vi "Serial.AML3.vi"(8 "error in":errorcluster, 10 "Serial Array":refnum<visa-resource-name>[](array[refnum])=["COM9", "COM8"], 11 "Data.PG":refnum<class "LV-Data.PGSQL.lvclass">) -> ()   [LabVIEW 2019, in "PGC2D.lvlib"]
uses:
  PGC2D.lvlib
  <userlib>/LevyLab/LV-Data/LV-Data.PG/LV-Data.PGSQL.lvclass
  sandbox/Instrument.AML.GetAll--Cluster.ctl
panel:
  out "Prep Status":string
  out "Analysis Status":string
  out "Prep Pressure (mbar)":dbl=4294966292.0
  out "Analysis Pressure (mbar)":dbl=4294966292.0
  out "Data.PG out":refnum<class "LV-Data.PGSQL.lvclass">
  out "timer (ms)":u32=4294966292
  in  "wait (ms)":u32=1000
  out "error out":errorcluster
  in  "OK":bool
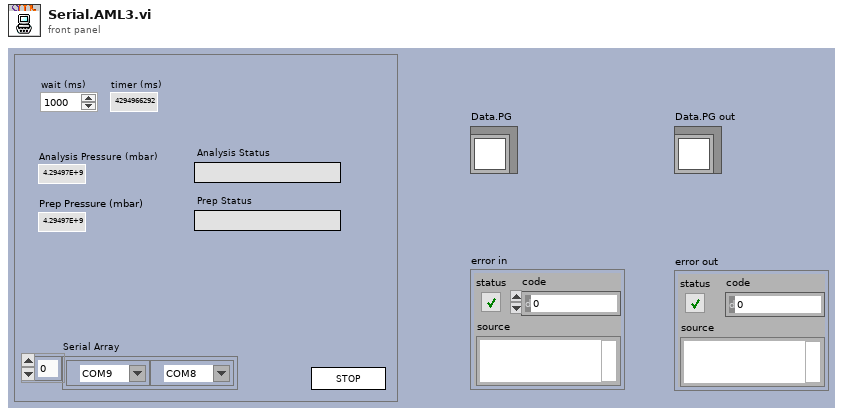
[diagram p1: front panel]
types:
  T1 = enum32{"Invalid", "Standard", "Closed", "Hidden", "Minimized", "Maximized"}
  T2 = enum32{"invalid app kind", "Development System", "Run Time System", "Student Edition", "Embedded LabVIEW", "Evaluation", "Custom"}
  T3 = typedef "Instrument.AML.GetAll--Cluster.ctl" = cluster{"IG Pressure (mbar)":dbl, "Pirani 1 Pressure (mbar)":dbl, "Pirani 2 Pressure (mbar)":dbl, "Emission Current (A)":dbl, "Trip A Pressure (mbar)":dbl, "Trip B Pressure (mbar)":dbl, "Trip C Pressure (mbar)":dbl, "Trip D Pressure (mbar)":dbl, "Instrument Status":string, "Fault":string, "Trip A Association":string, "Trip B Association":string, "Trip C Association":string, "Trip D Association":string, "Relay A":string, "Relay B":string, "Relay C":string, "Relay D":string}
  T4 = cluster{"Core":cluster{"Current VI Reference":refnum<vi>, "Close Panel on Exit?":bool}, "Data.PG":refnum<class "LV-Data.PGSQL.lvclass">, "Serial Array ":refnum<visa-resource-name>[], "AML cluster array":T3[], "Chamber ID":cluster{"Chamber name":string, "Trip pressure":dbl}[]}
  T5 = cluster{"Chamber name":string, "Trip pressure":dbl}[]
  T6 = cluster{"Current VI Reference":refnum<vi>, "Close Panel on Exit?":bool}
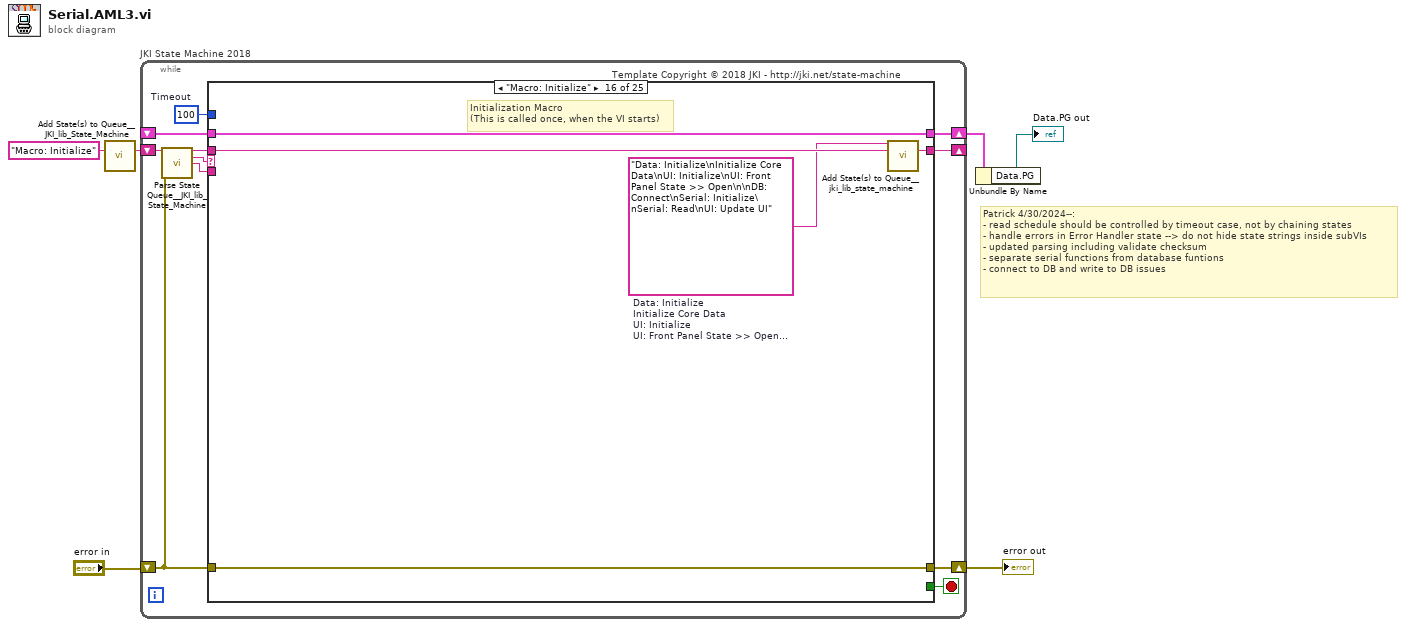
[diagram p0: block diagram]
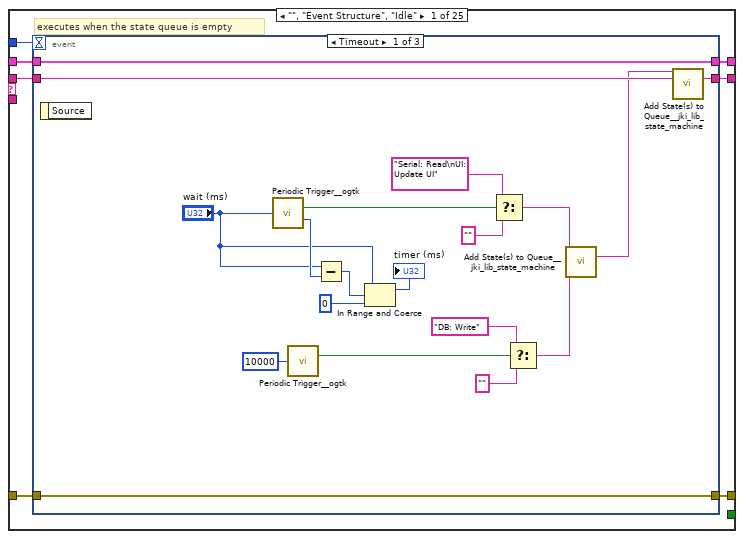
[diagram p2: hidden frame]
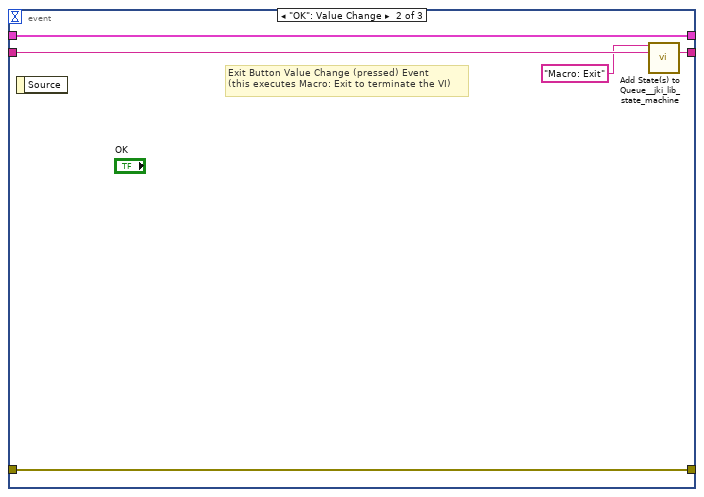
[diagram p3: hidden frame]
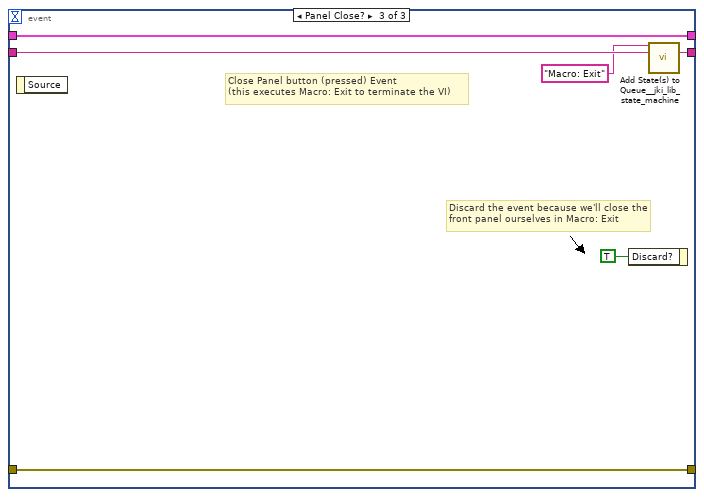
[diagram p4: hidden frame]
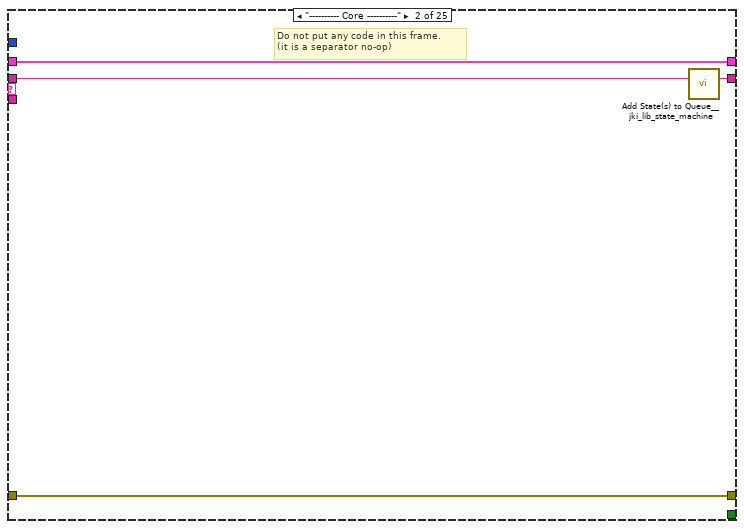
[diagram p5: hidden frame]
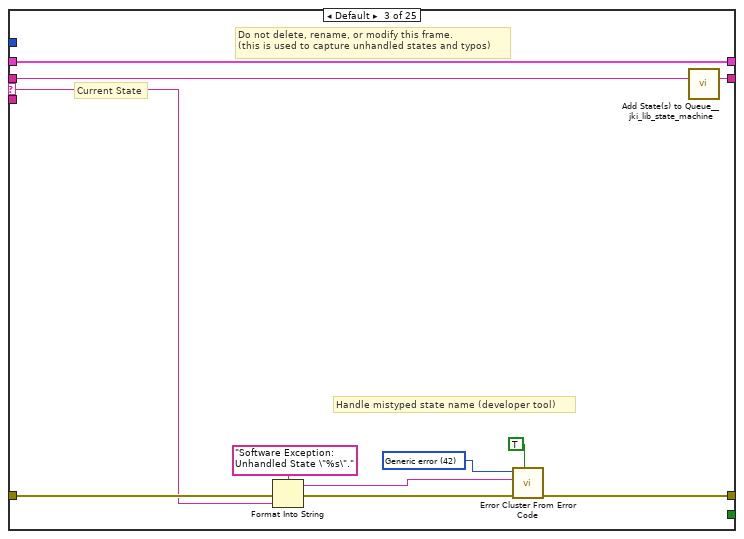
[diagram p6: hidden frame]
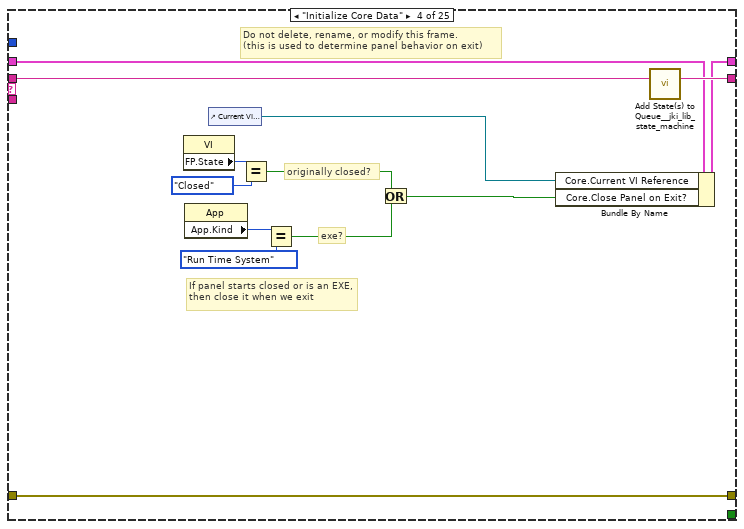
[diagram p7: hidden frame]
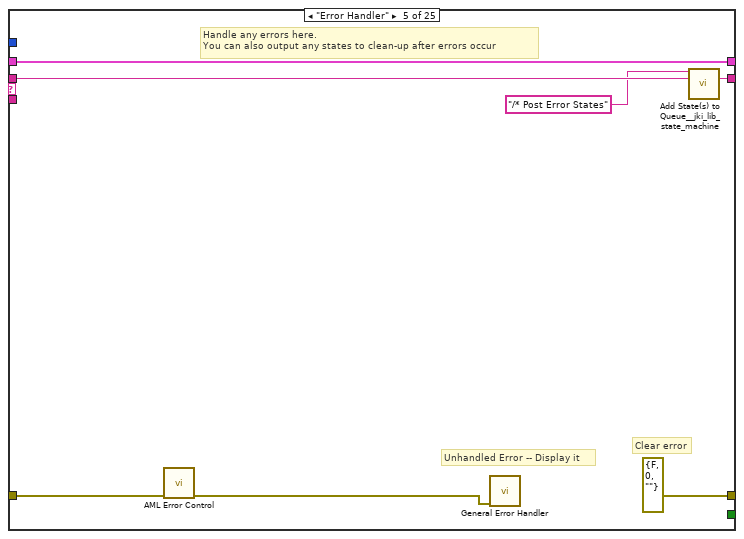
[diagram p8: hidden frame]
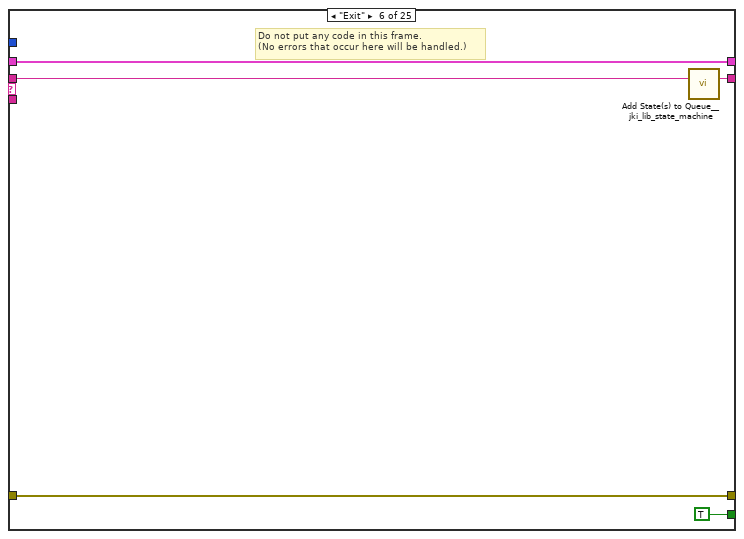
[diagram p9: hidden frame]
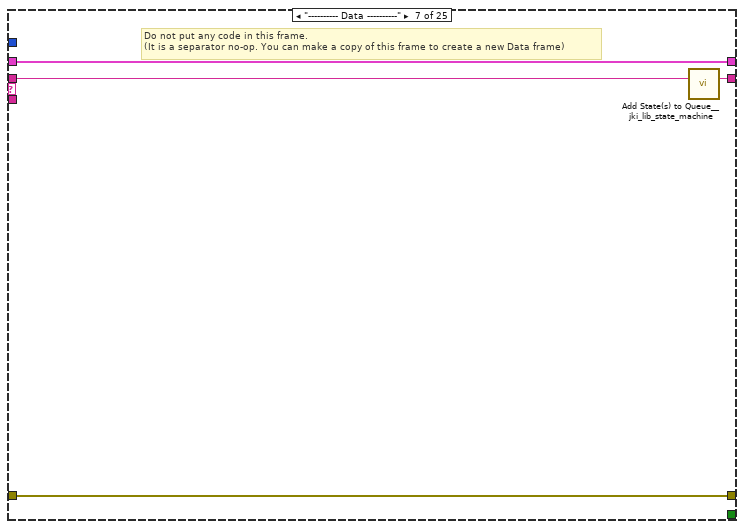
[diagram p10: hidden frame]
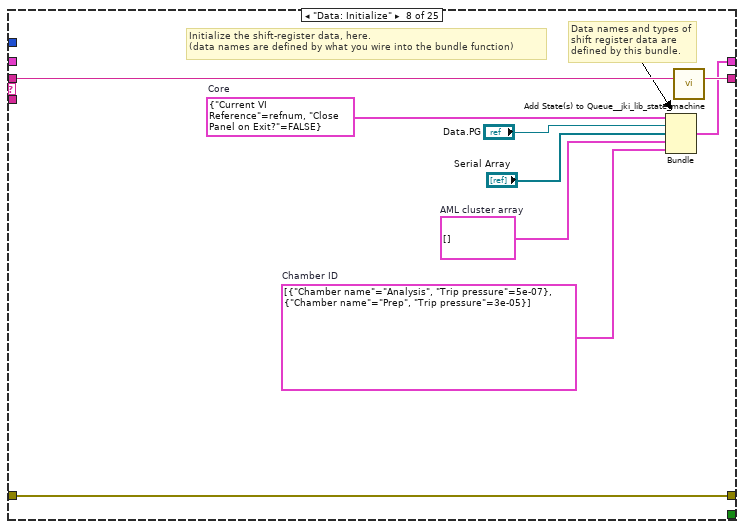
[diagram p11: hidden frame]
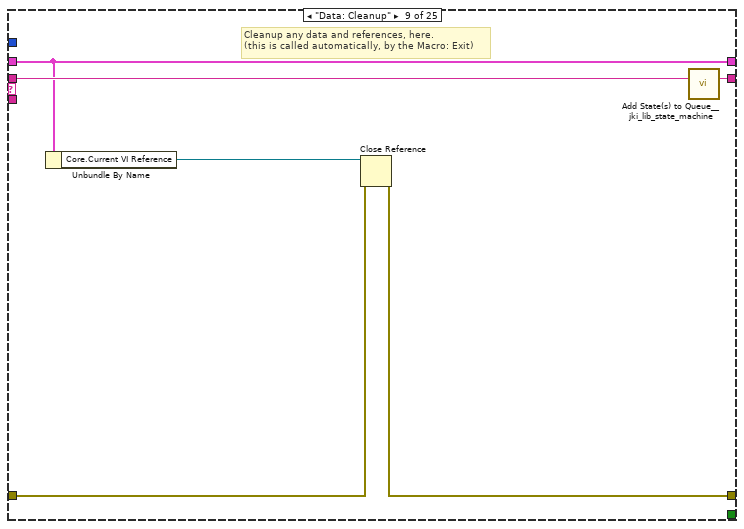
[diagram p12: hidden frame]
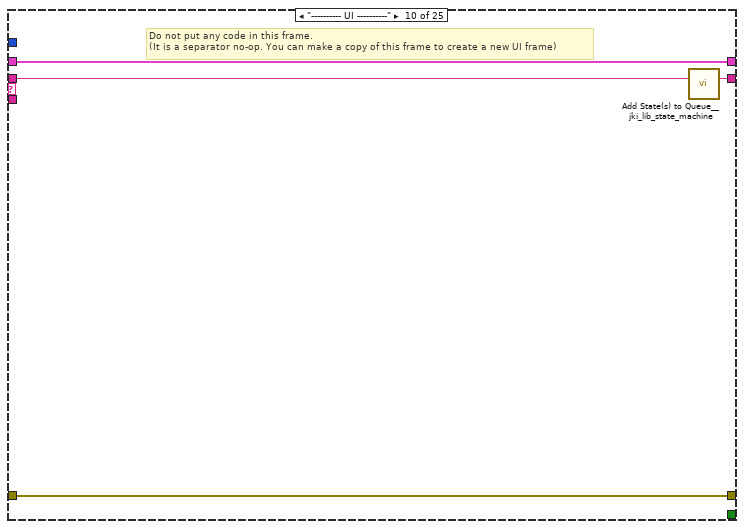
[diagram p13: hidden frame]
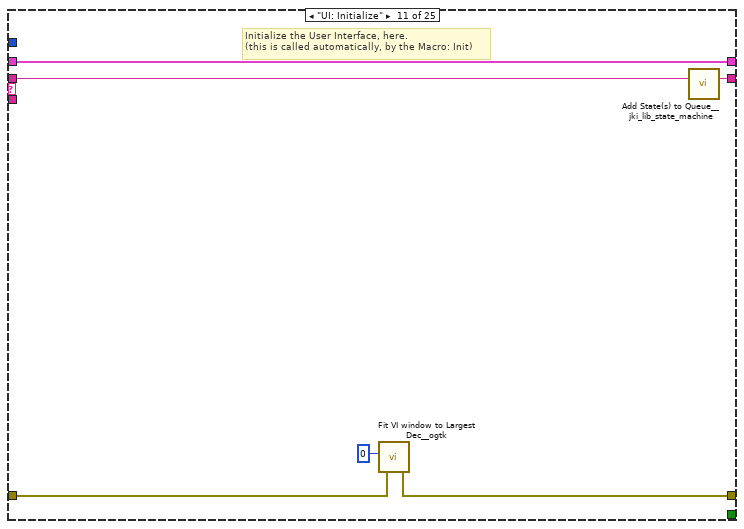
[diagram p14: hidden frame]
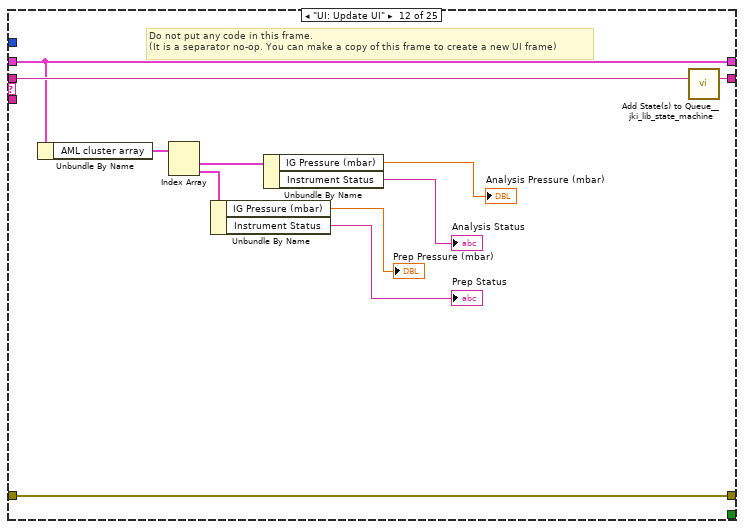
[diagram p15: hidden frame]
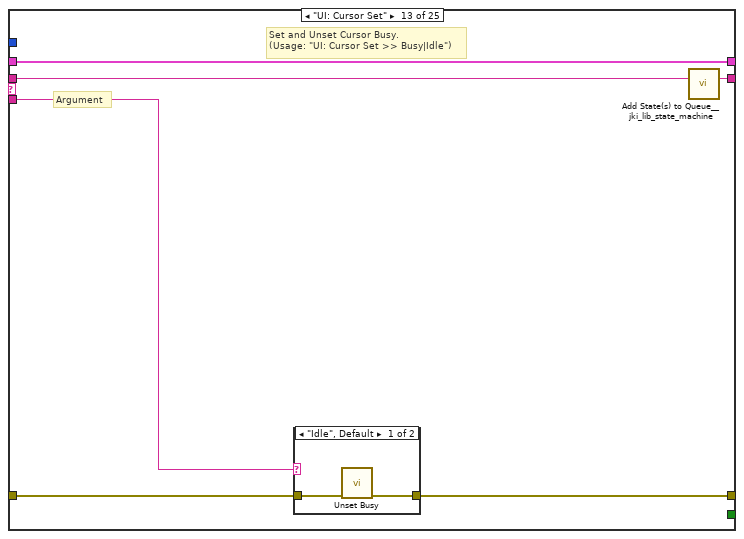
[diagram p16: hidden frame]
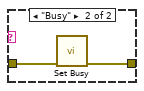
[diagram p17: hidden frame]
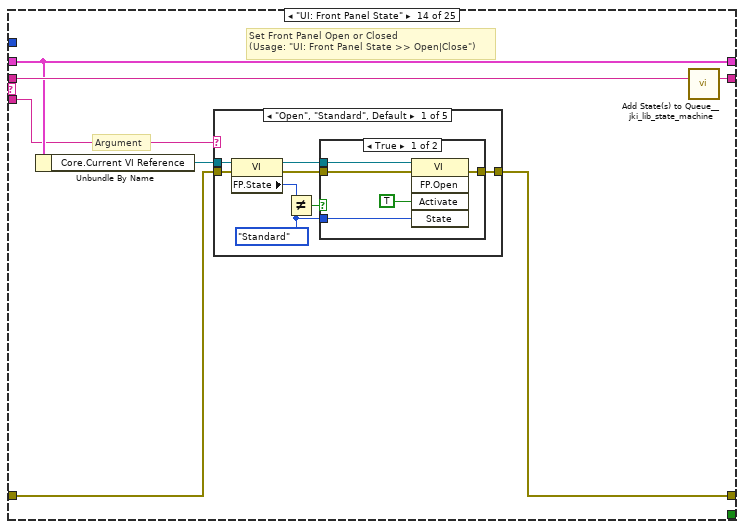
[diagram p18: hidden frame]
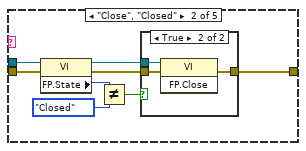
[diagram p20: hidden frame]
diagram:
  # "Patrick 4/30/2024--:\n- read schedule should be controlled by timeout case, not by chaining states\n- handle errors in Error Handler state --> do not hide state strings inside subVIs\n- updated parsing including validate checksum\n- separate serial functions from database funtions\n- connect to DB and write to DB issues"
  n1 = call <vilib>:"Add State(s) to Queue__JKI_lib_State_Machine.vi"("State(s) in (\"\")"="Macro: Initialize") -> ("States Out"=w6:string)  [unwired: 14 in]
  n2 = while "JKI State Machine 2018" {
    shift-right: [w10] -> w2
    shift-left: _ -> [w9]
    shift-right: [w13] -> w4
    shift-left: "error in" -> [w7]
    shift-right: [w12] -> _
    shift-left: w6 -> [w14]
    stop <- w11 stop-if-true
    w8 = 100  # Timeout
    # "Template Copyright © 2018 JKI - http://jki.net/state-machine"
    n3 = call <vilib>:"Parse State Queue__JKI_lib_State_Machine.vi"("State Queue"=w14, "Error In (no error)"=w7) -> ("Remaining States"=w16:string, "Current State"=w17:string, "Arguments"=w15:string)  [unwired: 11 in]
    n4 = case shown="\"Macro: Initialize\"" w17 {
      selector: w17 -> [_ _ w59 _ _ _ _ _ _ _ _ _ _ _ _ _ _ _ _ _ _ _ _ _ _]
      tunnel: w16 -> [w24 w58 w63 w82 w89 w94 w98 w107 w113 w117 w123 w134 w140 w151 w220 w225 w236 w240 w248 w262 w273 w282 w290 w295 w308]
      tunnel: w15 -> [_ _ _ _ _ _ _ _ _ _ _ _ w135 w145 _ _ _ _ _ _ _ _ _ _ _]
      tunnel: w9 -> [w22 w55 w61 w75 w83 w92 w95 _ w108 w114 w121 w131 w138 w147 w217 w222 w233 w237 w246 w255 w270 w279 w285 w292 w304]
      tunnel: [w21 w56 w65 w79 errorcluster {"status"=FALSE, "code"=0, "source"=""} ("error out") w91 w96 w104 w110 w115 w120 w132 w136 w148 w218 w223 w234 w238 w245 w254 w271 w280 w284 w298 w302] -> w13
      tunnel: w7 -> [w20 w56 w64 w79 w85 w91 w96 w104 w109 w115 w119 w132 w137 w149 w218 w223 w234 w238 w242 w258 w272 w280 w283 w299 w301]
      tunnel: [w23 w57 w62 w81 w88 w93 w97 w106 w112 w116 w122 w133 w139 w150 w219 w224 w235 w239 w247 w261 w274 w281 w289 w296 w307] -> w12
      tunnel: [_ _ _ _ _ TRUE _ _ _ _ _ _ _ _ _ _ _ _ _ _ _ _ _ _ _] -> w11
      tunnel: [w19 w55 w61 w80 w83 w92 w95 w105 w108 w114 w121 w131 w138 w147 w217 w222 w233 w237 w241 w256 w270 w279 w286 w294 w305] -> w10
      tunnel: w8 -> [w18 _ _ _ _ _ _ _ _ _ _ _ _ _ _ _ _ _ _ _ _ _ _ _ _]
      frame "", "Event Structure", "Idle" {
        # "executes when the state queue is empty"
        n5 = event shown="[0] Timeout" {
          selector: _ -> [_ _ _]
          dyn-events: _ -> [_ _ _]
          timeout: w18 -> [_ _ _]
          tunnel: w24 -> [w43 w48 w54]
          tunnel: [w42 w47 w53] -> w23
          tunnel: w22 -> [w40 w45 w51]
          tunnel: [w41 w46 w52] -> w21
          tunnel: w20 -> [w41 w46 w52]
          tunnel: [w40 w45 w51] -> w19
          event Timeout {
            n6 = event-data() -> ()  [unwired: 1 in, 1 out]
            n7 = call <userlib>:"Periodic Trigger__ogtk.vi"("time (ms)"="wait (ms)") -> ("Triggered"=w38:bool, "timer value"=w39:u32)  [unwired: 12 in, 1 out]
            n8 = call <userlib>:"Periodic Trigger__ogtk.vi"("time (ms)"=u32 10000) -> ("Triggered"=w31:bool)  [unwired: 12 in, 2 out]
            n9 = Subtract(x="wait (ms)", y=w39) -> (x-y=w27:u32)
            n10 = In Range and Coerce(upper limit="wait (ms)", x=w27, lower limit=u32 0) -> (coerced(x)=→"timer (ms)":u32)  [unwired: 1 out]
            n11 = Select(t="Serial: Read\nUI: Update UI" ("State(s) in Front (\"\")"), s=w38, f="" ("State(s) in Front (\"\")")) -> (s? t:f=w35:string)
            n12 = Select(t="DB: Write" ("State(s) in Front (\"\")"), s=w31, f="" ("State(s) in Front (\"\")")) -> (s? t:f=w30:string)
            n13 = call <vilib>:"Add State(s) to Queue__jki_lib_state_machine.vi"("State(s) in Front (\"\")"=w35, "State(s) at Back (\"\")"=w30) -> ("States Out"=w29:string)  [unwired: 13 in]
            n14 = call <vilib>:"Add State(s) to Queue__jki_lib_state_machine.vi"("State(s) in Front (\"\")"=w29, "State(s) in (\"\")"=w43) -> ("States Out"=w42:string)  [unwired: 13 in]
          }
          event "OK": Value Change {
            # "Exit Button Value Change (pressed) Event\n(this executes Macro: Exit to terminate the VI)"
            n15 = event-data() -> ()  [unwired: 1 in, 1 out]
            n16 = call <vilib>:"Add State(s) to Queue__jki_lib_state_machine.vi"("State(s) in Front (\"\")"="Macro: Exit", "State(s) in (\"\")"=w48) -> ("States Out"=w47:string)  [unwired: 13 in]
          }
          event Panel Close? {
            # "Discard the event because we'll close the front panel ourselves in Macro: Exit"
            # "Close Panel button (pressed) Event\n(this executes Macro: Exit to terminate the VI)"
            n17 = event-data() -> ()  [unwired: 1 in, 1 out]
            n18 = event-data("Discard?"=TRUE) -> ()  [unwired: 1 in, 1 out]
            n19 = call <vilib>:"Add State(s) to Queue__jki_lib_state_machine.vi"("State(s) in Front (\"\")"="Macro: Exit", "State(s) in (\"\")"=w54) -> ("States Out"=w53:string)  [unwired: 13 in]
          }
        }
      }
      frame "---------- Core ----------" {
        # "Do not put any code in this frame.\n(it is a separator no-op)"
        n20 = call <vilib>:"Add State(s) to Queue__jki_lib_state_machine.vi"("State(s) in (\"\")"=w58) -> ("States Out"=w57:string)  [unwired: 14 in]
      }
      frame Default {
        w68 = 42 items=["No error", "Argument error", "Memory is full", "Out of zone", "End of file", "File already open", "Generic file I/O error", "File not found", "File permission error", "Disk is full", "Duplicate path", "Too many files open", "System feature not enabled", "Resource file not found", "Cannot add resource", "Resource not found", "Image not found", "Image memory error", "Pen does not exist", "Config type invalid", "Config token not found", "Config parse error", "Config memory error", "Bad external code format", "Bad external code offset", "External code not present", "Null window", "Destroy window error", "Null menu", "Print aborted", "Bad print record", "Print driver error", "Windows error during printing", "Memory error during printing", "Print dialog error", "Generic print error", "Invalid device refnum", "Device not found", "Device parameter error", "Device unit error", "Cannot open device", "Device call aborted", "Generic error", "Cancelled by user", "Object ID too low", "Object ID too high", "Object not in heap", "Unknown heap", "Unknown object (invalid DefProc)", "Unknown object (DefProc not in table)", "Message out of range", "Invalid (null) method", "Unknown message", "Manager call not supported", "Bad address", "Network operation in progress", "Network operation timed out", "Connection is busy", "Network attribute not supported", "Network error", "Address in use", "System out of memory", "Connection aborted", "Connection refused", "Not connected", "Already connected", "Connection closed", "Initialization error (interapplication manager)", "Bad occurrence", "Wait on unbound occurrence handler", "Occurrence queue overflow", "Datalog type conflict", "Unused", "Unrecognized type (interapplication manager)", "Memory corrupt", "Failed to make temporary DLL", "Old CIN version", "Drag socket not found", "Failed to load drop-object", "Failed to register OLE object", "Failed to release OLE object", "Format specifier type mismatch", "Unknown format specifier", "Too few format specifiers", "Too many format specifiers", "Scan failed", "Newer CIN version", "Error converting to variant", "Runtime menu error", "Password tampered", "Variant attribute not found", "Incompatible variant data type", "Event data is not available", "Event Store is not present", "Occurrence is not found", "Event Queue is not created", "Event info is not available", "Refnum passed is NULL", "Error retrieving Class GUID", "Error retrieving CoClass GUID", "Error retrieving TypeLib GUID.", "Bad built application magic bytes.", "Specific driver is different from the specific driver associated with the Logical Name.", "There is no session opened to the class driver.", "Max Error", "MAX - Error with config objects", "MAX - Error loading configuration", "MAX - Group not supported"]
        # "Current State"
        # "Do not delete, rename, or modify this frame.\n(this is used to capture unhandled states and typos)"
        # "Handle mistyped state name (developer tool)"
        n21 = Format Into String(format string="Software Exception: Unhandled State \"%s\"." ("message"), error in=w64, w59) -> (resulting string=w67:string, error out=w66:errorcluster)  [unwired: 1 in]
        n22 = call <vilib>:"Error Cluster From Error Code.vi"("show call chain? (False)"=TRUE, "error in (no error)"=w66, "error message (\"\")"=w67, "error code (0)"=w68) -> ("error out"=w65:errorcluster)  [unwired: 5 in]
        n23 = call <vilib>:"Add State(s) to Queue__jki_lib_state_machine.vi"("State(s) in (\"\")"=w63) -> ("States Out"=w62:string)  [unwired: 14 in]
      }
      frame "Initialize Core Data" {
        # "Do not delete, rename, or modify this frame.\n(this is used to determine panel behavior on exit)"
        # "originally closed?"
        # "exe?"
        # "If panel starts closed or is an EXE, then close it when we exit"
        n24 = property class="VI"() -> ("FP.State"=w72:T1)  [unwired: 2 in, 2 out]
        n25 = property class="App"() -> ("App.Kind"=w78:T2)  [unwired: 2 in, 2 out]
        n26 = control-ref of="Current VI Reference"() -> (w73:refnum<vi>)
        n27 = Equal?(x=w72, y=T1."Closed" ("Front Panel Window:State")) -> (x = y?=w70:bool)
        n28 = Equal?(x=w78, y=T2."Run Time System" ("Application:Kind")) -> (x = y?=w76:bool)
        n29 = Or(x=w70, y=w76) -> (x .or. y?=w74:bool)
        n30 = Bundle By Name(cluster=w75, "Core.Current VI Reference"=w73, "Core.Close Panel on Exit?"=w74) -> (w80:T4)
        n31 = call <vilib>:"Add State(s) to Queue__jki_lib_state_machine.vi"("State(s) in (\"\")"=w82) -> ("States Out"=w81:string)  [unwired: 14 in]
      }
      frame "Error Handler" {
        # "Unhandled Error -- Display it"
        # "Handle any errors here.\nYou can also output any states to clean-up after errors occur"
        # "Clear error"
        n32 = call "AML Error Control.vi"("input cluster"=w85) -> ("error out"=w84:errorcluster)  [unwired: 8 in, 2 out]
        n33 = call <vilib>:"General Error Handler.vi"("error in (no error)"=w84) -> ()  [unwired: 10 in, 5 out]
        n34 = call <vilib>:"Add State(s) to Queue__jki_lib_state_machine.vi"("State(s) in Front (\"\")"="/* Post Error States", "State(s) in (\"\")"=w89) -> ("States Out"=w88:string)  [unwired: 13 in]
      }
      frame "Exit" {
        # "Do not put any code in this frame.\n(No errors that occur here will be handled.)"
        n35 = call <vilib>:"Add State(s) to Queue__jki_lib_state_machine.vi"("State(s) in (\"\")"=w94) -> ("States Out"=w93:string)  [unwired: 14 in]
      }
      frame "---------- Data ----------" {
        # "Do not put any code in this frame.\n(It is a separator no-op. You can make a copy of this frame to create a new Data frame)"
        n36 = call <vilib>:"Add State(s) to Queue__jki_lib_state_machine.vi"("State(s) in (\"\")"=w98) -> ("States Out"=w97:string)  [unwired: 14 in]
      }
      frame "Data: Initialize" {
        w100 = T5 [{"Chamber name"="Analysis", "Trip pressure"=5e-07}, {"Chamber name"="Prep", "Trip pressure"=3e-05}]  # Chamber ID
        w101 = T3[] []  # AML cluster array
        w103 = T6 {"Current VI Reference"=refnum, "Close Panel on Exit?"=FALSE}  # Core
        # "Data names and types of shift register data are defined by this bundle."
        # "Initialize the shift-register data, here.\n(data names are defined by what you wire into the bundle function)"
        n37 = Bundle("Core"=w103, "Data.PG"="Data.PG", "Serial Array"="Serial Array", "AML cluster array"=w101, "Chamber ID"=w100) -> (w105:T4)  [unwired: 1 in]
        n38 = call <vilib>:"Add State(s) to Queue__jki_lib_state_machine.vi"("State(s) in (\"\")"=w107) -> ("States Out"=w106:string)  [unwired: 14 in]
      }
      frame "Data: Cleanup" {
        # "Cleanup any data and references, here.\n(this is called automatically, by the Macro: Exit)"
        n39 = Unbundle By Name(w108) -> ("Core.Current VI Reference"=w111:refnum<vi>)
        n40 = Close Reference(reference=w111, error in (no error)=w109) -> (error out=w110:errorcluster)
        n41 = call <vilib>:"Add State(s) to Queue__jki_lib_state_machine.vi"("State(s) in (\"\")"=w113) -> ("States Out"=w112:string)  [unwired: 14 in]
      }
      frame "---------- UI ----------" {
        # "Do not put any code in this frame.\n(It is a separator no-op. You can make a copy of this frame to create a new UI frame)"
        n42 = call <vilib>:"Add State(s) to Queue__jki_lib_state_machine.vi"("State(s) in (\"\")"=w117) -> ("States Out"=w116:string)  [unwired: 14 in]
      }
      frame "UI: Initialize" {
        # "Initialize the User Interface, here.\n(this is called automatically, by the Macro: Init)"
        n43 = call <userlib>:"Fit VI window to Largest Dec__ogtk.vi"("error in (no error)"=w119, "border spacing (2 px)"=0) -> ("error out"=w120:errorcluster)  [unwired: 4 in, 1 out]
        n44 = call <vilib>:"Add State(s) to Queue__jki_lib_state_machine.vi"("State(s) in (\"\")"=w123) -> ("States Out"=w122:string)  [unwired: 14 in]
      }
      frame "UI: Update UI" {
        # "Do not put any code in this frame.\n(It is a separator no-op. You can make a copy of this frame to create a new UI frame)"
        n45 = Unbundle By Name(w131) -> ("AML cluster array"=w130:T3[])
        n46 = Index Array(array=w130) -> (element #1=w129:T3, element #2=w128:T3)  [unwired: 2 in]
        n47 = Unbundle By Name(w128) -> ("IG Pressure (mbar)"=→"Prep Pressure (mbar)":dbl, "Instrument Status"=→"Prep Status":string)
        n48 = Unbundle By Name(w129) -> ("IG Pressure (mbar)"=→"Analysis Pressure (mbar)":dbl, "Instrument Status"=→"Analysis Status":string)
        n49 = call <vilib>:"Add State(s) to Queue__jki_lib_state_machine.vi"("State(s) in (\"\")"=w134) -> ("States Out"=w133:string)  [unwired: 14 in]
      }
      frame "UI: Cursor Set" {
        # "Argument"
        # "Set and Unset Cursor Busy.\n(Usage: \"UI: Cursor Set >> Busy|Idle\")"
        n50 = case shown="\"Idle\", Default" w135 {
          tunnel: w137 -> [w142 w144]
          tunnel: [w141 w143] -> w136
          frame "Idle", Default {
            n51 = call <vilib>:"Unset Busy.vi"("error in (no error)"=w142) -> ("error out"=w141:errorcluster)  [unwired: 10 in]
          }
          frame "Busy" {
            n52 = call <vilib>:"Set Busy.vi"("error in (no error)"=w144) -> ("error out"=w143:errorcluster)  [unwired: 9 in, 1 out]
          }
        }
        n53 = call <vilib>:"Add State(s) to Queue__jki_lib_state_machine.vi"("State(s) in (\"\")"=w140) -> ("States Out"=w139:string)  [unwired: 14 in]
      }
      frame "UI: Front Panel State" {
        # "Argument"
        # "Set Front Panel Open or Closed\n(Usage: \"UI: Front Panel State >> Open|Close\")"
        n54 = Unbundle By Name(w147) -> ("Core.Current VI Reference"=w146:refnum<vi>)
        n55 = case shown="\"Open\", \"Standard\", Default" w145 {
          tunnel: w149 -> [w157 w172 w183 w196 w209]
          tunnel: [w159 w173 w185 w198 w211] -> w148
          tunnel: w146 -> [w158 w170 w184 w197 w210]
          frame "Open", "Standard", Default {
            w152 = T1."Standard" ("State")
            n56 = property class="VI"(reference=w158, error in=w157) -> (reference out=w155:refnum<vi>, error out=w156:errorcluster, "FP.State"=w154:T1)
            n57 = Not Equal?(x=w154, y=w152) -> (x != y?=w153:bool)
            n58 = case shown="True" w153 {
              tunnel: [w163 w165] -> w159
              tunnel: w156 -> [w162 w165]
              tunnel: w155 -> [w161 _]
              tunnel: w152 -> [w160 _]
              frame True {
                n59 = invoke class="VI" method="FP.Open"(reference=w161, error in=w162, "Activate"=TRUE, "State"=w160) -> (error out=w163:errorcluster)  [unwired: 1 in, 4 out]
              }
              frame False {
              }
            }
          }
          frame "Close", "Closed" {
            n60 = property class="VI"(reference=w170, error in=w172) -> (reference out=w169:refnum<vi>, error out=w171:errorcluster, "FP.State"=w167:T1)
            n61 = Not Equal?(x=w167, y=T1."Closed" ("Front Panel Window:State")) -> (x != y?=w166:bool)
            n62 = case shown="True" w166 {
              tunnel: [w174 w177] -> w173
              tunnel: w171 -> [w174 w176]
              tunnel: w169 -> [_ w175]
              frame False {
              }
              frame True {
                n63 = invoke class="VI" method="FP.Close"(reference=w175, error in=w176) -> (error out=w177:errorcluster)  [unwired: 1 in, 2 out]
              }
            }
          }
          frame "Hidden", "Hide" {
            w178 = T1."Hidden" ("State")
            n64 = property class="VI"(reference=w184, error in=w183) -> (reference out=w181:refnum<vi>, error out=w182:errorcluster, "FP.State"=w180:T1)
            n65 = Not Equal?(x=w180, y=w178) -> (x != y?=w179:bool)
            n66 = case shown="True" w179 {
              tunnel: [w189 w190] -> w185
              tunnel: w182 -> [w188 w190]
              tunnel: w181 -> [w187 _]
              tunnel: w178 -> [w186 _]
              frame True {
                n67 = invoke class="VI" method="FP.Open"(reference=w187, error in=w188, "State"=w186) -> (error out=w189:errorcluster)  [unwired: 2 in, 4 out]
              }
              frame False {
              }
            }
          }
          frame "Minimize", "Minimized" {
            w191 = T1."Minimized" ("State")
            n68 = property class="VI"(reference=w197, error in=w196) -> (reference out=w194:refnum<vi>, error out=w195:errorcluster, "FP.State"=w193:T1)
            n69 = Not Equal?(x=w193, y=w191) -> (x != y?=w192:bool)
            n70 = case shown="True" w192 {
              tunnel: [w202 w203] -> w198
              tunnel: w195 -> [w201 w203]
              tunnel: w194 -> [w200 _]
              tunnel: w191 -> [w199 _]
              frame True {
                n71 = invoke class="VI" method="FP.Open"(reference=w200, error in=w201, "State"=w199) -> (error out=w202:errorcluster)  [unwired: 2 in, 4 out]
              }
              frame False {
              }
            }
          }
          frame "Maximize", "Maximized" {
            w204 = T1."Maximized" ("State")
            n72 = property class="VI"(reference=w210, error in=w209) -> (reference out=w207:refnum<vi>, error out=w208:errorcluster, "FP.State"=w206:T1)
            n73 = Not Equal?(x=w206, y=w204) -> (x != y?=w205:bool)
            n74 = case shown="True" w205 {
              tunnel: [w215 w216] -> w211
              tunnel: w208 -> [w214 w216]
              tunnel: w207 -> [w213 _]
              tunnel: w204 -> [w212 _]
              frame True {
                n75 = invoke class="VI" method="FP.Open"(reference=w213, error in=w214, "State"=w212) -> (error out=w215:errorcluster)  [unwired: 2 in, 4 out]
              }
              frame False {
              }
            }
          }
        }
        n76 = call <vilib>:"Add State(s) to Queue__jki_lib_state_machine.vi"("State(s) in (\"\")"=w151) -> ("States Out"=w150:string)  [unwired: 14 in]
      }
      frame "---------- Macro ----------" {
        # "Do not put any code in this frame.\n(It is a separator no-op. You can make a copy of this frame to create a new Macro frame)"
        n77 = call <vilib>:"Add State(s) to Queue__jki_lib_state_machine.vi"("State(s) in (\"\")"=w220) -> ("States Out"=w219:string)  [unwired: 14 in]
      }
      frame "Macro: Initialize" {
        w221 = "Data: Initialize\nInitialize Core Data\nUI: Initialize\nUI: Front Panel State >> Open\n\nDB: Connect\nSerial: Initialize\nSerial: Read\nUI: Update UI"  # Data: Initialize Initialize Core Data UI: Initialize UI: Front Panel State >> Open  DB: Connect Serial: Initialize Serial: Read UI: Update UI
        # "Initialization Macro\n(This is called once, when the VI starts)"
        n78 = call <vilib>:"Add State(s) to Queue__jki_lib_state_machine.vi"("State(s) in Front (\"\")"=w221, "State(s) in (\"\")"=w225) -> ("States Out"=w224:string)  [unwired: 13 in]
      }
      frame "Macro: Exit" {
        # "Exit Macro\n(This is called once, when the VI exits)"
        n79 = Unbundle By Name(w233) -> ("Core.Close Panel on Exit?"=w232:bool)
        n80 = Select(t="UI: Front Panel State >> Close", s=w232, f="") -> (s? t:f=w229:string)
        n81 = call <vilib>:"Add State(s) to Queue__jki_lib_state_machine.vi"("State(s) in Front (\"\")"="Serial: Close\nDB: Disconnect", "State(s) in (\"\")"=w229, "State(s) at Back (\"\")"="Data: Cleanup\nExit") -> ("States Out"=w227:string)  [unwired: 12 in]
        n82 = call <vilib>:"Add State(s) to Queue__jki_lib_state_machine.vi"("State(s) in Front (\"\")"=w227, "State(s) in (\"\")"=w236) -> ("States Out"=w235:string)  [unwired: 13 in]
      }
      frame "---------- Serial ----------" {
        # "Template Separator\n(You can make a copy of, or modify, this frame)"
        n83 = call <vilib>:"Add State(s) to Queue__jki_lib_state_machine.vi"("State(s) in (\"\")"=w240) -> ("States Out"=w239:string)  [unwired: 14 in]
      }
      frame "Serial: Initialize" {
        n84 = Unbundle By Name(w246) -> ("Serial Array"=w244:refnum<visa-resource-name>[])
        n85 = for {
          tunnel: w244 -> [w252] mode=indexing
          tunnel: [w251] -> w243 mode=indexing
          tunnel: w242 -> [w250]
          tunnel: [w249] -> w245
          n86 = call "Initialize Serial.vi"("error in (no error)"=w250, "VISA resource name"=w252) -> ("error out"=w249:errorcluster, "VISA resource name out"=w251:refnum<visa-resource-name>)  [unwired: 8 in]
        }
        n87 = Bundle By Name(cluster=w246, "Serial Array"=w243) -> (w241:T4)
        n88 = call <vilib>:"Add State(s) to Queue__jki_lib_state_machine.vi"("State(s) in (\"\")"=w248) -> ("States Out"=w247:string)  [unwired: 14 in]
      }
      frame "Serial: Read" {
        n89 = Unbundle By Name(w255) -> ("Serial Array"=w259:refnum<visa-resource-name>[])
        n90 = for {
          tunnel: [w269] -> w260 mode=indexing
          tunnel: w259 -> [w268] mode=indexing
          tunnel: [w267] -> w253 mode=indexing
          tunnel: w258 -> [w264]
          tunnel: [w266] -> w254
          n91 = call <userlib>:"Wait (ms)__ogtk.vi"("error in (no error)"=w264, "milliseconds to wait"=u32 250) -> ("error out"=w265:errorcluster)  [unwired: 8 in, 1 out]
          n92 = call "Read Serial.vi"("error in (no error)"=w265, "VISA Reference"=w268) -> ("error out"=w266:errorcluster, "GetAll"=w267:T3, "VISA Reference out"=w269:refnum<visa-resource-name>)  [unwired: 7 in]
        }
        n93 = Bundle By Name(cluster=w255, "Serial Array"=w260, "AML cluster array"=w253) -> (w256:T4)
        n94 = call <vilib>:"Add State(s) to Queue__jki_lib_state_machine.vi"("State(s) in Front (\"\")"="", "State(s) in (\"\")"=w262) -> ("States Out"=w261:string)  [unwired: 13 in]
      }
      frame "Serial: Close" {
        n95 = Unbundle By Name(w270) -> ("Serial Array"=w275:refnum<visa-resource-name>[])
        n96 = for {
          tunnel: w275 -> [w278] mode=indexing
          tunnel: w272 -> [w277]
          tunnel: [w276] -> w271
          n97 = call "Close Serial.vi"("error in (no error)"=w277, "VISA Reference"=w278) -> ("error out"=w276:errorcluster)  [unwired: 9 in]
        }
        n98 = call <vilib>:"Add State(s) to Queue__jki_lib_state_machine.vi"("State(s) in (\"\")"=w273) -> ("States Out"=w274:string)  [unwired: 14 in]
      }
      frame "---------- DB ----------" {
        # "Template Separator\n(You can make a copy of, or modify, this frame)"
        n99 = call <vilib>:"Add State(s) to Queue__jki_lib_state_machine.vi"("State(s) in (\"\")"=w282) -> ("States Out"=w281:string)  [unwired: 14 in]
      }
      frame "DB: Connect" {
        # "Template Separator\n(You can make a copy of, or modify, this frame)"
        n100 = Unbundle By Name(w285) -> ("Data.PG"=w288:refnum<class "LV-Data.PGSQL.lvclass">)
        n101 = call <userlib>:"PGSQL.Open.vi"("error in (no error)"=w283, "Data.PG in"=w288) -> ("error out"=w284:errorcluster, "Data.PG out"=w287:refnum<class "LV-Data.PGSQL.lvclass">)  [unwired: 8 in]
        n102 = Bundle By Name(cluster=w285, "Data.PG"=w287) -> (w286:T4)
        n103 = call <vilib>:"Add State(s) to Queue__jki_lib_state_machine.vi"("State(s) in (\"\")"=w290) -> ("States Out"=w289:string)  [unwired: 14 in]
      }
      frame "DB: Write" {
        n104 = Unbundle By Name(w292) -> ("Data.PG"=w300:refnum<class "LV-Data.PGSQL.lvclass">, "AML cluster array"=w293:T3[], "Chamber ID"=w291:T5)
        n105 = call "Serial Write to DB.vi"("error in"=w299, "Chamber ID"=w291, "AML Cluster const"=w293, "Data.PG in"=w300) -> ("error out"=w298:errorcluster, "Data.PG out"=w297:refnum<class "LV-Data.PGSQL.lvclass">)  [unwired: 4 in, 2 out]
        n106 = Bundle By Name(cluster=w292, "Data.PG"=w297) -> (w294:T4)
        n107 = call <vilib>:"Add State(s) to Queue__jki_lib_state_machine.vi"("State(s) in (\"\")"=w295) -> ("States Out"=w296:string)  [unwired: 14 in]
      }
      frame "DB: Disconnect" {
        # "Template Separator\n(You can make a copy of, or modify, this frame)"
        n108 = Unbundle By Name(w304) -> ("Data.PG"=w303:refnum<class "LV-Data.PGSQL.lvclass">)
        n109 = call-dynamic "Close.vi"("error in (no error)"=w301, "Data.PG in"=w303) -> ("error out"=w302:errorcluster, "Data.PG out"=w306:refnum<class "LV-Data.PGSQL.lvclass">)  [unwired: 8 in]
        n110 = Bundle By Name(cluster=w304, "Data.PG"=w306) -> (w305:T4)
        n111 = call <vilib>:"Add State(s) to Queue__jki_lib_state_machine.vi"("State(s) in (\"\")"=w308) -> ("States Out"=w307:string)  [unwired: 14 in]
      }
    }
  }
  "error out" <- w4
  n112 = Unbundle By Name(w2) -> ("Data.PG"=→"Data.PG out":refnum<class "LV-Data.PGSQL.lvclass">)
